vi "DMA.Write Multiple.vi"(8 "error in (no error)":errorcluster, 9 "timeout ms per transfer (1000)":u32=1000, 10 "DMA Transfer Specs":T1[](array[typedef]) {"Block Descriptors"."next descriptor ptr" format="%08x"; "Block Descriptors"."data size" format="%08x"; "Block Descriptors"."data ptr (upper)" format="%08x"; "Block Descriptors"."data ptr (lower)" format="%08x"; "Block Descriptors"."descriptor ptr (aligned)" format="%08x"; "Block Descriptors"."descriptor size" format="%08x"; "Block Descriptors"."descriptor ptr (VISA)" format="%08x"; "RFM Address" format="%08x"}, 11 "GE 5565PIORC":refnum<class "GE 5565PIORC.lvclass">) -> (0 "error out":errorcluster, 1 "Timed out?":bool, 2 "DMA Transfer Specs out":T1[](array[typedef]) {"Block Descriptors"."next descriptor ptr" format="%08x"; "Block Descriptors"."data size" format="%08x"; "Block Descriptors"."data ptr (upper)" format="%08x"; "Block Descriptors"."data ptr (lower)" format="%08x"; "Block Descriptors"."descriptor ptr (aligned)" format="%08x"; "Block Descriptors"."descriptor size" format="%08x"; "Block Descriptors"."descriptor ptr (VISA)" format="%08x"; "RFM Address" format="%08x"}, 3 "GE 5565PIORC out":refnum<class "GE 5565PIORC.lvclass">)   [LabVIEW 2016, in "GE 5565PIORC.lvclass"]
uses:
  GE 5565PIORC.lvclass
  Controls/DMA Transfer Spec.ctl
  Controls/DMA Block Descriptor.ctl
  GE 5565PIORC.lvclass/GE 5565PIORC.ctl
  DMA.Start Transfer.vi
  DMA.Wait for Done Interrupt Event.vi
  Interrupts/Discard PXI Interrupt Events.vi
  DMA.Configure.vi
  Registers/Local Configuration.DMACSR0.DMA Start.Set.vi
  Interrupts/Wait for PXI Interrupt Events.vi
  Registers/Local Configuration.DMACSR0.DMA Clear Interrupt.Set.vi
  <vilib>/Utility/error.llb/Clear Errors.vi
  DMA.Transfer Size.vi
  Registers/Local Configuration.PCI Address.Set.vi
  Registers/Local Configuration.DMADPR0.First Descriptor Address.Set.vi
  DMA.Scatter-Gather.Link Block Descriptors.vi
  DMA.Scatter-Gather.Commit Blocks.vi
  Registers/Local Configuration.Local Address.Set.vi
  Registers/Local Configuration.Transfer Size.Set.vi
  Registers/Local Configuration.DMADPR0.Transfer Direction.Set.vi
  Registers/Local Configuration.DMAMODE0.Scatter-Gather Enable.Set.vi
  Binary Operations/Set Bits.vi
  Binary Operations/Set Bits U32.vi
  Registers/Local Configuration.Get Register Offset.vi
  Binary Operations/Get Bits.vi
  Binary Operations/Get Bits U32.vi
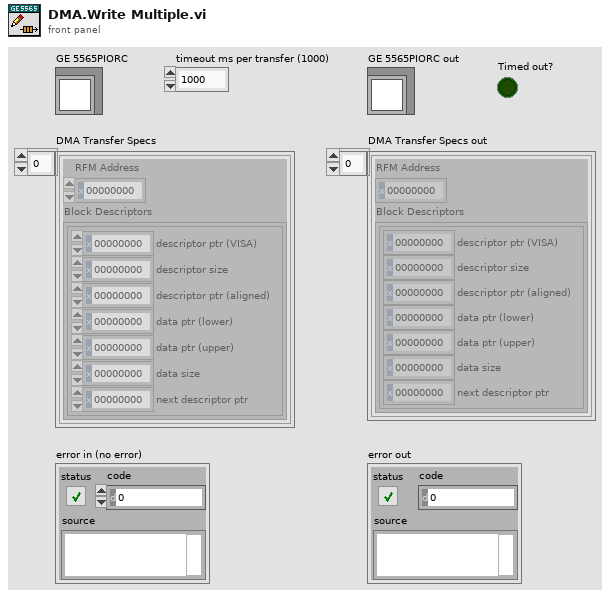
[diagram p1: front panel]
types:
  T1 = typedef "GE 5565PIORC.lvclass/DMA Transfer Spec.ctl" = cluster{"RFM Address":u32, "Block Descriptors":T2[]}
  T2 = typedef "GE 5565PIORC.lvclass/DMA Block Descriptor.ctl" = cluster{"descriptor ptr (VISA)":u32, "descriptor size":u32, "descriptor ptr (aligned)":u32, "data ptr (lower)":u32, "data ptr (upper)":u32, "data size":u32, "next descriptor ptr":u32}
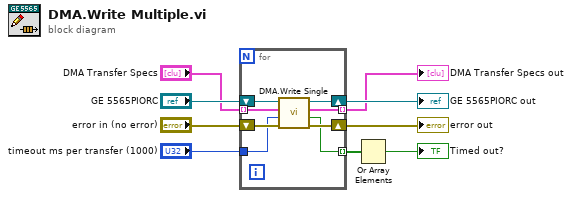
[diagram p0: block diagram]
diagram:
  n1 = for {
    shift-right: [w14] -> w6
    shift-left: "error in (no error)" -> [w17]
    shift-right: [w15] -> w7
    shift-left: "GE 5565PIORC" -> [w16]
    tunnel: "DMA Transfer Specs" -> [w13] mode=indexing
    tunnel: [w12] -> w5 mode=indexing
    tunnel: "timeout ms per transfer (1000)" -> [w10]
    tunnel: [w11] -> w3 mode=indexing
    n2 = call "DMA.Write Single.vi"("error in (no error)"=w17, "timeout ms (1000)"=w10, "DMA Transfer Spec"=w13, "GE 5565PIORC"=w16) -> ("error out"=w14:errorcluster, "Timed out?"=w11:bool, "DMA Transfer Spec out"=w12:T1, "GE 5565PIORC out"=w15:refnum<class "GE 5565PIORC.lvclass">)  [unwired: 4 in]
  }
  "error out" <- w6
  "GE 5565PIORC out" <- w7
  "DMA Transfer Specs out" <- w5
  n3 = Or Array Elements(Boolean array=w3) -> (logical OR=→"Timed out?":bool)
